vi "Enqueue Message.vi"(8 "error in":errorcluster, 11 "Message Data":T1) -> (0 "error out":errorcluster)   [LabVIEW 2015, in "Generic Module Library.lvlib" / "Template G_Module.lvlib"]
uses:
  Template G_Module.lvlib
  Queue Support/Queue Reference Actions.ctl
  Private Controls/Module Message Cluster Components/Acknowledge Data Cluster.ctl
  Private Controls/Module Message Cluster.ctl
  Private Controls/Module Message Cluster Components/Message Data Cluster.ctl
  Private Controls/Module Message Cluster Components/Ack Payload.ctl
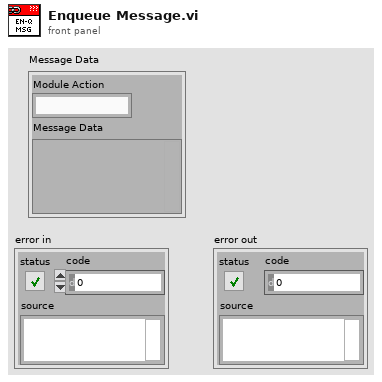
[diagram p1: front panel]
types:
  T1 = typedef "Generic Module Library.lvlib/Template G_Module.lvlib/Message Data Cluster.ctl" = cluster{"Module Action":string, "Message Data":variant}
  T2 = typedef "Generic Module Library.lvlib/Template G_Module.lvlib/Acknowledge Data Cluster.ctl" = cluster{"Ack Requested":bool, "Ack Notifier Ref":refnum<notifier>, "Response Payload":T3}
  T3 = typedef "Generic Module Library.lvlib/Template G_Module.lvlib/Ack Payload.ctl" = cluster{"Response Data":string, "error out":errorcluster}
  T4 = typedef "Generic Module Library.lvlib/Template G_Module.lvlib/Module Message Cluster.ctl" = cluster{"Message Data":T1, "Acknowledge Data":T2}
  T5 = typedef "Generic Module Library.lvlib/Template G_Module.lvlib/Queue Reference Actions.ctl" = enum16{"Release", "Set", "Get"}
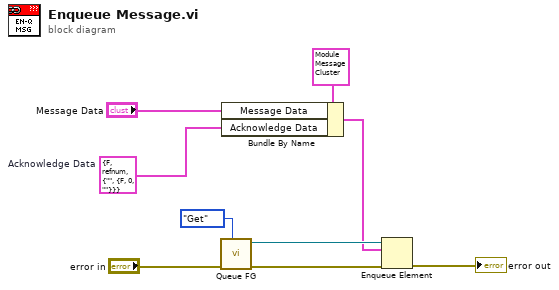
[diagram p0: block diagram]
diagram:
  w1 = T2 {"Ack Requested"=FALSE, "Ack Notifier Ref"=refnum, "Response Payload"={"Response Data"="", "error out"={"status"=FALSE, "code"=0, "source"=""}}}  # Acknowledge Data
  n1 = call "Queue FG.vi"("Queue Reference Actions"=Queue_Reference_Actions."Get", "error in"="error in") -> ("error out"=w7:errorcluster, "Queue out"=w6:refnum<queue>)  [unwired: 8 in]
  n2 = Bundle By Name(cluster=T4 {"Message Data"={"Module Action"="", "Message Data"=variant}, "Acknowledge Data"={"Ack Requested"=FALSE, "Ack Notifier Ref"=refnum, "Response Payload"={"Response Data"="", "error out"={"status"=FALSE, "code"=0, "source"=""}}}} ("element"), "Message Data"="Message Data", "Acknowledge Data"=w1) -> (w2:T4)
  n3 = Enqueue Element(queue=w6, element=w2, error in (no error)=w7) -> (error out=→"error out":errorcluster)  [unwired: 1 in, 2 out]
